vi "Generate_I2C.vi"(8 "Error_In":errorcluster, 10 "Mode":T1, 11 "7Bit_Address_In":refnum<class "7 Bit Address.lvclass">) -> (0 "Error_Out":errorcluster, 3 "7Bit_Address_Out":refnum<class "7 Bit Address.lvclass">)   [LabVIEW 2023, in "7 Bit Address.lvclass"]
uses:
  7 Bit Address.lvclass
  D:/Git/Assignments/SDLC_I2C/SDLC_I2C_LV23V/Class/I2C/I2C.lvclass
  Controls/Mode.ctl
  Controls/I2C_States.ctl
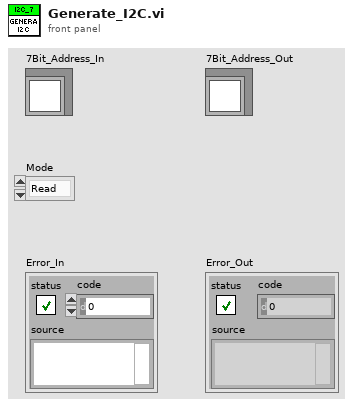
[diagram p1: front panel]
types:
  T1 = typedef "Mode.ctl" = enum16{"Read", "Write"}
  T2 = typedef "I2C_States.ctl" = enum16{"Start", "Byte", "Ack_Nack", "Stop"}
  T3 = typedef "Converted_Data.ctl" = cluster{"Vmin":dbl, "Vmax":dbl, "Input":string, "Off_Set (uS)":dbl, "T_HD_STA (uS)":dbl, "Sample_Per_Us":dbl, "T_HD_DAT (uS)":dbl, "T_SU_DAT (uS)":dbl, "Frequency (kHz)":dbl, "T_SU_STO":dbl, "T_Off (uS)":dbl, "T_On (uS)":dbl, "T_BUF":dbl, "Target_Address":u16, "Selected_Register_Address":u8, "Byte_Array":u8[], "Target_Name":string, "Register_Name":string[], "Register_Address":u8[], "Ring":T4}
  T4 = typedef "Menu_Ring.ctl" = u16
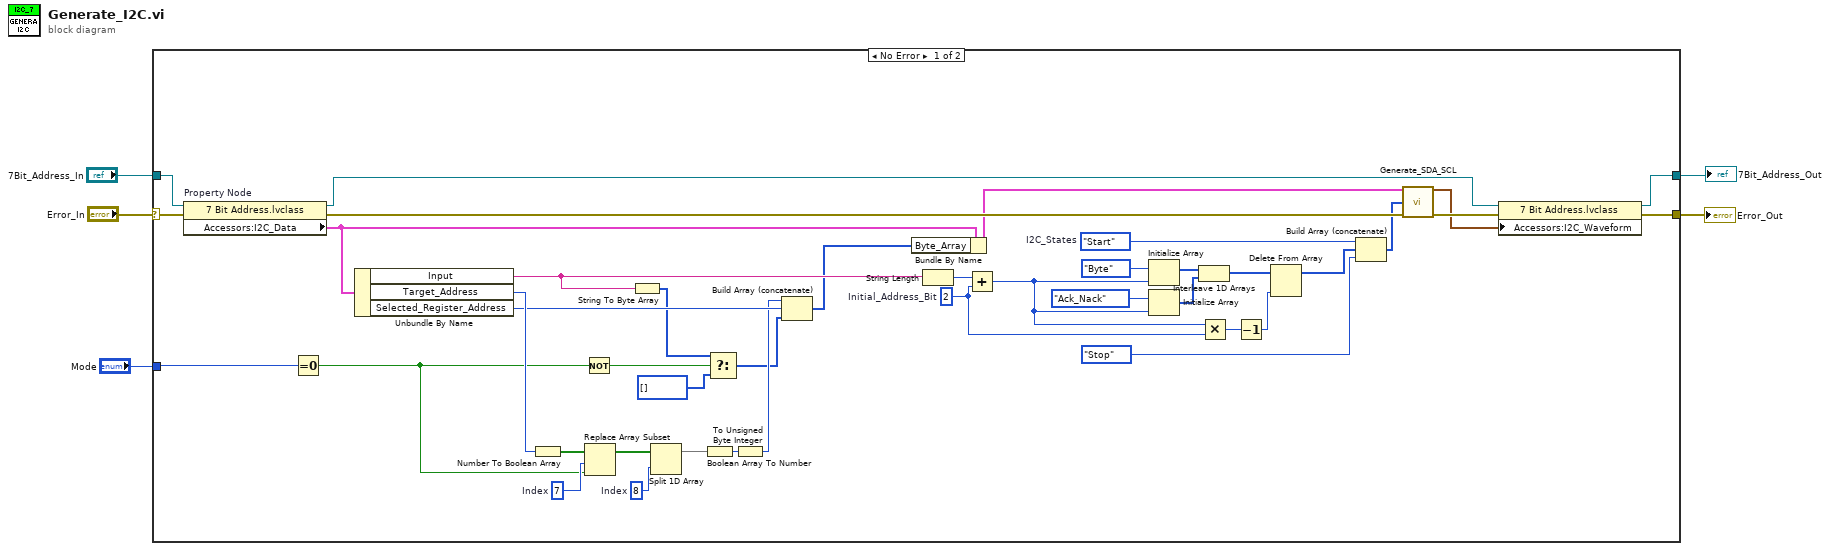
[diagram p0: block diagram]
diagram:
  n1 = case shown="No Error" "Error_In" {
    selector: "Error_In" -> [w45 w48]
    tunnel: [w24 w48] -> w5
    tunnel: [w25 w47] -> w4
    tunnel: "7Bit_Address_In" -> [w36 w47]
    tunnel: "Mode" -> [w32 _]
    frame No Error {
      w10 = 2  # Initial_Address_Bit
      w21 = 8  # Index
      w30 = 7  # Index
      w43 = I2C_States."Start"  # I2C_States
      n2 = property on="Property Node" class="7 Bit Address.lvclass"(reference=w36, error in=w45) -> (reference out=w35:refnum<class "7 Bit Address.lvclass">, error out=w44:errorcluster, "Accessors:I2C_Data"=w15:T3)
      n3 = Equal To 0?(x=w32) -> (x = 0?=w16:bool)
      n4 = Unbundle By Name(w15) -> ("Input"=w33:string, "Target_Address"=w29:u16, "Selected_Register_Address"=w27:u8)
      n5 = Number To Boolean Array(number=w29) -> (Boolean array=w31:bool[])
      n6 = Not(x=w16) -> (.not. x?=w20:bool)
      n7 = Replace Array Subset(array=w31, new element=w16, index=w30) -> (w23:bool[])
      n8 = String To Byte Array(string=w33) -> (unsigned byte array=w19:u8[])
      n9 = Split 1D Array(array=w23, index=w21) -> (first subarray=w22:bool[])  [unwired: 1 out]
      n10 = Boolean Array To Number(Boolean array=w22) -> (number=w28:u32)
      n11 = Select(t=w19, s=w20, f=u8[] []) -> (s? t:f=w18:u8[])
      n12 = To Unsigned Byte Integer(number=w28) -> (unsigned 8bit integer=w26:u8)
      n13 = Build Array (concatenate)(w26, w27, w18) -> (w13:u8[])
      n14 = Bundle By Name(cluster=w15, "Byte_Array"=w13) -> (w14:T3)
      n15 = String Length(string=w33) -> (length=w12:i32)
      n16 = Add(x=w12, y=w10) -> (x+y=w11:i32)
      n17 = Initialize Array(I2C_States."Byte" ("Enum"), w11) -> (w40:T2[])
      n18 = Initialize Array(I2C_States."Ack_Nack" ("element"), w11) -> (w39:T2[])
      n19 = Interleave 1D Arrays(w40, w39) -> (w8:T2[])
      n20 = Multiply(x=w11, y=w10) -> (x*y=w9:i32)
      n21 = Decrement(x=w9) -> (x-1=w6:i32)
      n22 = Delete From Array(array=w8, index=w6) -> (array with subset deleted=w7:T2[])  [unwired: 1 in, 1 out]
      n23 = Build Array (concatenate)(w43, w7, I2C_States."Stop" ("element")) -> (w37:T2[])
      n24 = call "Generate_SDA_SCL.vi"("Data"=w14, "Data_Sequence"=w37, "Error_In"=w44) -> ("Waveform Graph"=w34:waveform(dbl)[], "Error_Out"=w46:errorcluster)  [unwired: 11 in]
      n25 = property class="7 Bit Address.lvclass"(reference=w35, error in=w46, "Accessors:I2C_Waveform"=w34) -> (reference out=w25:refnum<class "7 Bit Address.lvclass">, error out=w24:errorcluster)
    }
    frame Error {
    }
  }
  "Error_Out" <- w5
  "7Bit_Address_Out" <- w4
